vi "KB-CalNewC.vi"(6 "offset Y":sgl=4.0, 7 "Matches (Geometric Matching 1)":T1[](array[typedef]) {"Correlation Score" format="%.2f"; "Target Template Curve Score" format="%.2f"; "Template Target Curve Score" format="%.2f"; "Bounding Box"."y" format="%.2f"; "Bounding Box"."x" format="%.2f"; "Position"."y" format="%.2f"; "Position"."x" format="%.2f"; "Score" format="%.2f"; "Scale" format="%.2f"; "Angle" format="%.2f"; "Occlusion %" format="%.2f"}, 8 "內环半径":i32=16, 9 "Outer Radius":i32=10, 10 "I roi":T2 {"Contours"."Type" items=["No Selection", "Point", "Line", "Rectangle", "Oval", "Polygon", "Freehand Region", "Annulus", "Unused2", "Unused3", "Broken Line", "Freehand Line", "Rotated Rectangle"]}, 11 "Fitted Circle (Find Circular Edge 1)":T3 {"Average SNR (dB)" format="%.2f"; "Average Strength" format="%.2f"; "Roundness (Real-World)" format="%.2f"; "Radius (Real-World)" format="%.2f"; "Center (Real-World)"."Y" format="%.2f"; "Center (Real-World)"."X" format="%.2f"; "Radius (Pixels)" format="%.2f"; "Center (Pixels)"."Y" format="%.2f"; "Center (Pixels)"."X" format="%.2f"}) -> (3 "ROI Descriptor":T2 {"Contours"."Type" items=["No Selection", "Point", "Line", "Rectangle", "Oval", "Polygon", "Freehand Region", "Annulus", "Unused2", "Unused3", "Broken Line", "Freehand Line", "Rotated Rectangle"]})   [LabVIEW 2015]
uses:
  <vilib>/vision/Pattern Matching.llb/IMAQ GM Match Report.ctl
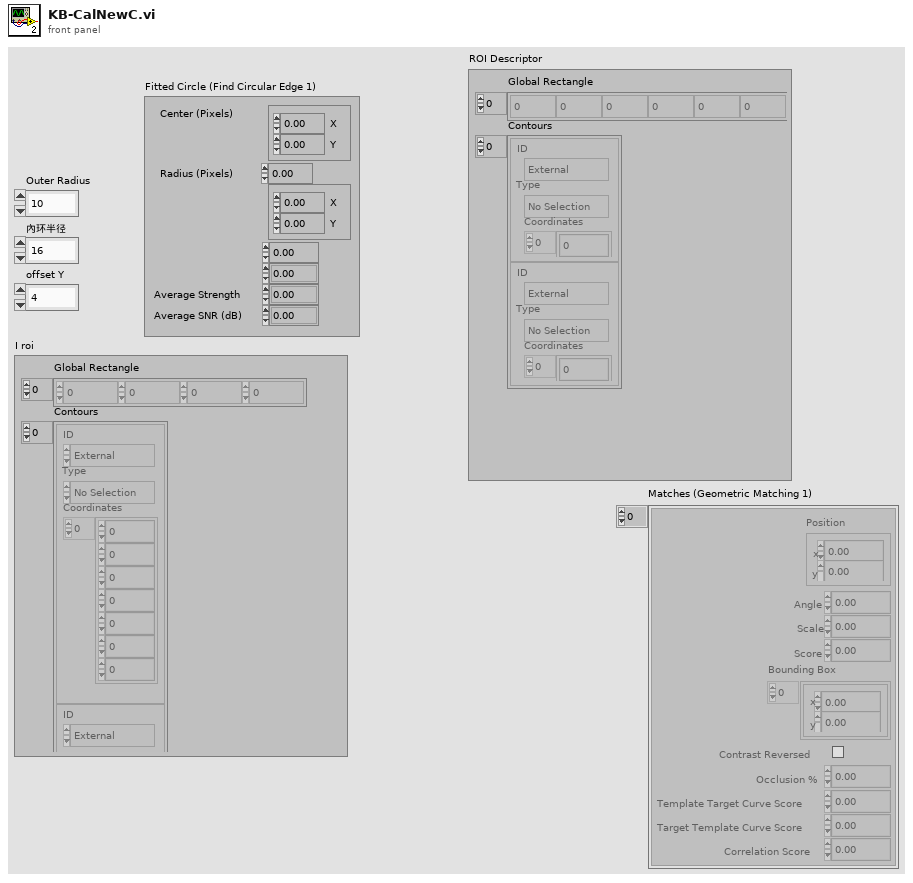
[diagram p1: front panel]
types:
  T1 = typedef "IMAQ GM Match Report.ctl" = cluster{"Position":cluster{"x":sgl, "y":sgl}, "Angle":sgl, "Scale":sgl, "Score":sgl, "Bounding Box":cluster{"x":sgl, "y":sgl}[], "Contrast Reversed":bool, "Occlusion %":sgl, "Template Target Curve Score":sgl, "Target Template Curve Score":sgl, "Correlation Score":sgl}
  T2 = typedef "ROI Descriptor" = cluster{"Global Rectangle":i32[], "Contours":cluster{"ID":enum32{"External", "Internal"}, "Type":u32, "Coordinates":i32[]}[]}
  T3 = cluster{"Center (Pixels)":cluster{"X":sgl, "Y":sgl}, "Radius (Pixels)":dbl, "Center (Real-World)":cluster{"X":sgl, "Y":sgl}, "Radius (Real-World)":dbl, "Roundness (Real-World)":dbl, "Average Strength":dbl, "Average SNR (dB)":dbl}
  T4 = typedef "IMAQ Circle" = cluster{"Center X":i32, "Center Y":i32, "Inner Radius":i32, "Outer Radius":i32, "Start Angle":dbl, "End Angle":dbl}
  T5 = cluster{"ID":enum32{"External", "Internal"}, "Type":u32, "Coordinates":i32[]}[]
  T6 = cluster{"ID":enum32{"External", "Internal"}, "Type":u32, "Coordinates":i32[]}
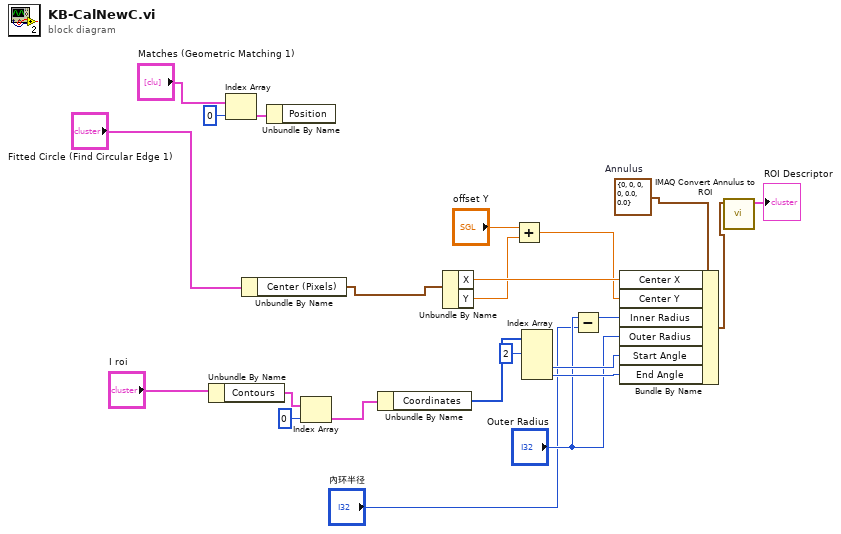
[diagram p0: block diagram]
diagram:
  w22 = T4 {"Center X"=0, "Center Y"=0, "Inner Radius"=0, "Outer Radius"=0, "Start Angle"=0.0, "End Angle"=0.0}  # Annulus
  n1 = Unbundle By Name("I roi") -> ("Contours"=w19:T5)
  n2 = Index Array(array="Matches (Geometric Matching 1)", index=0 ("索引")) -> (element=w2:T1)
  n3 = Unbundle By Name("Fitted Circle (Find Circular Edge 1)") -> ("Center (Pixels)"=w1:cluster{"X":sgl, "Y":sgl})
  n4 = Unbundle By Name(w2) -> ()  [unwired: 1 out]
  n5 = Index Array(array=w19, index=0 ("索引")) -> (element=w17:T6)
  n6 = Unbundle By Name(w17) -> ("Coordinates"=w16:i32[])
  n7 = Unbundle By Name(w1) -> ("X"=w21:sgl, "Y"=w7:sgl)
  n8 = Add(x="offset Y", y=w7) -> (x+y=w5:sgl)
  n9 = Index Array(array=w16, index #1=2 ("索引")) -> (element #3=w14:i32, element #4=w13:i32)  [unwired: 3 in, 2 out]
  n10 = Subtract(x="Outer Radius", y="內环半径") -> (x-y=w8:i32)
  n11 = Bundle By Name(cluster=w22, "Center X"=w21, "Center Y"=w5, "Inner Radius"=w8, "Outer Radius"="Outer Radius", "Start Angle"=w14, "End Angle"=w13) -> (w11:T4)
  n12 = call "IMAQ Convert Annulus to ROI"("Annulus"=w11) -> ("ROI Descriptor"=→"ROI Descriptor":T2)  [unwired: 8 in, 1 out]
